vi "Main_flow_full_mqtt_correct.vi"() -> ()   [LabVIEW 2022 SP3]
uses:
  D:/UOM/EE2044 - Electrical Measurements and Instrumentation/Project/Measurment Project/Quaxo_MQTT_LabVIEW-master/Controls/Connection_Return_Codes.ctl
  D:/UOM/EE2044 - Electrical Measurements and Instrumentation/Project/Measurment Project/Quaxo_MQTT_LabVIEW-master/Controls/QoS.ctl
  D:/UOM/EE2044 - Electrical Measurements and Instrumentation/Project/Measurment Project/Quaxo_MQTT_LabVIEW-master/Controls/Retain_Flag.ctl
  D:/UOM/EE2044 - Electrical Measurements and Instrumentation/Project/Measurment Project/Quaxo_MQTT_LabVIEW-master/Controls/DUP_Flag.ctl
  D:/UOM/EE2044 - Electrical Measurements and Instrumentation/Project/Measurment Project/Quaxo_MQTT_LabVIEW-master/Controls/Connect_Flags.ctl
  D:/UOM/EE2044 - Electrical Measurements and Instrumentation/Project/Measurment Project/Quaxo_MQTT_LabVIEW-master/Controls/User_Info.ctl
  <vilib>/DAQmx/write.llb/DAQmx Write (Digital Bool 1Line 1Point).vi
  <vilib>/DAQmx/read.llb/DAQmx Read (Digital Bool 1Line 1Point).vi
  <vilib>/DAQmx/read.llb/DAQmx Read (Analog 1D DBL NChan 1Samp).vi
  <vilib>/DAQmx/create/channels.llb/DAQmx Create Channel (AI-Voltage-Basic).vi
  <vilib>/DAQmx/create/channels.llb/DAQmx Create Channel (DO-Digital Output).vi
  <vilib>/DAQmx/create/channels.llb/DAQmx Create Channel (DI-Digital Input).vi
  <vilib>/DAQmx/miscellaneous.llb/DAQmx Fill In Error Info.vi
  D:/UOM/EE2044 - Electrical Measurements and Instrumentation/Project/Measurment Project/Quaxo_MQTT_LabVIEW-master/MQTT_Functions.lvlib
panel:
  out "?":bool
  out "?":bool
  out "?":bool
  in  "stop 2":bool
  in  "Publish Meta":cluster{"QoS":T1, "Retain":T2, "DUP":T3}
  out "Connection Status":T4=enum."Connection refused: not authorized"
  in  "MQTT Broker":cluster{"address (IP)":string, "port":u16}={"address (IP)"="broker.mqttdashboard.com", "port"=1883}
  in  "Client ID":string="NodeE-12345"
  out "main loop executed":dbl
  out "Servo Angle":dbl(knob) scale=0.0..150.0
  in  "stop (F)":bool
  out "PWM Wave":dynamicdata(graph) caption="Square"
  in  "Frequency":dbl=50.0
  in  "Offset":dbl=2.5
  in  "Amplitude":dbl=2.5
  out "LDR Value":dbl(knob) scale=0.0..10.0
  in  "Relay 2":tag
  in  "Relay 1":tag
  in  "UP DOWN 2":tag
  in  "UP DOWN 1":tag
  in  "Buzzer":tag
  out "Counter":dbl
  out "OUT COUNT":dbl
  out "IN COUNT":dbl
  in  "Door IR 1 & 2 & LDR":tag
  in  "Trigger Period(sec)":dbl
  out "Current Time":dbl
  in  "Mode":dbl
  in  "stop":bool
  # "Light Mode"
  # "Dev1/ai4:6"
  # "Low"
  # "Medium"
  # "High"
  # "Dev1/port0/line2"
  # "This Indicate the status of light mode in the room"
  # "Dev1/port0/line0"
  # "Dev1/port0/line1"
  # "Dev1/port0/line3"
  # "Dev1/port0/line4"
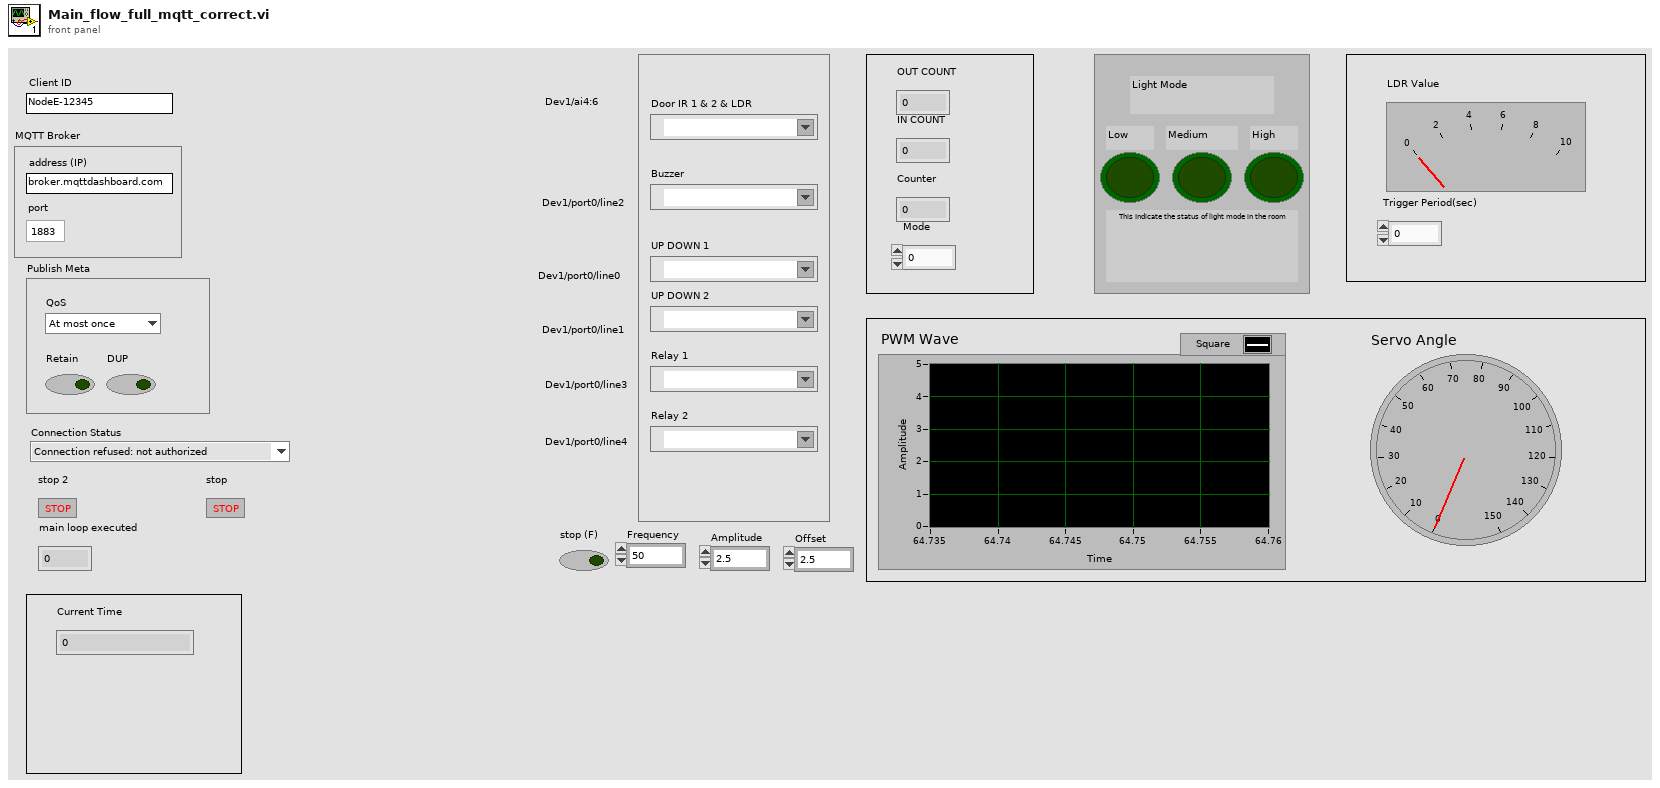
[diagram p1: front panel]
types:
  T1 = typedef "MQTT_Functions.lvlib/QoS.ctl" = enum8{"At most once", "At least once", "Exactly once", "Reserved"}
  T2 = typedef "MQTT_Functions.lvlib/Retain_Flag.ctl" = bool
  T3 = typedef "MQTT_Functions.lvlib/DUP_Flag.ctl" = bool
  T4 = typedef "MQTT_Functions.lvlib/Connection_Return_Codes.ctl" = enum16{"Connection accepted", "Connection refused: unacceptable protocol version", "Connection refused: identifier rejected", "Connection refused: Server unavailable", "Connection refused: bad user name or password", "Connection refused: not authorized"}
  T5 = typedef "MQTT_Functions.lvlib/User_Info.ctl" = cluster{"User Name":string, "Password":string}
  T6 = typedef "MQTT_Functions.lvlib/Connect_Flags.ctl" = cluster{"user name":bool, "password":bool, "will retain":bool, "will flag":bool, "clean session":bool, "reserved":bool, "will QoS":T1}
  T7 = cluster{"QoS":T1, "DUP":T3, "Retain":T2, "Keep Alive (sec)":u16}
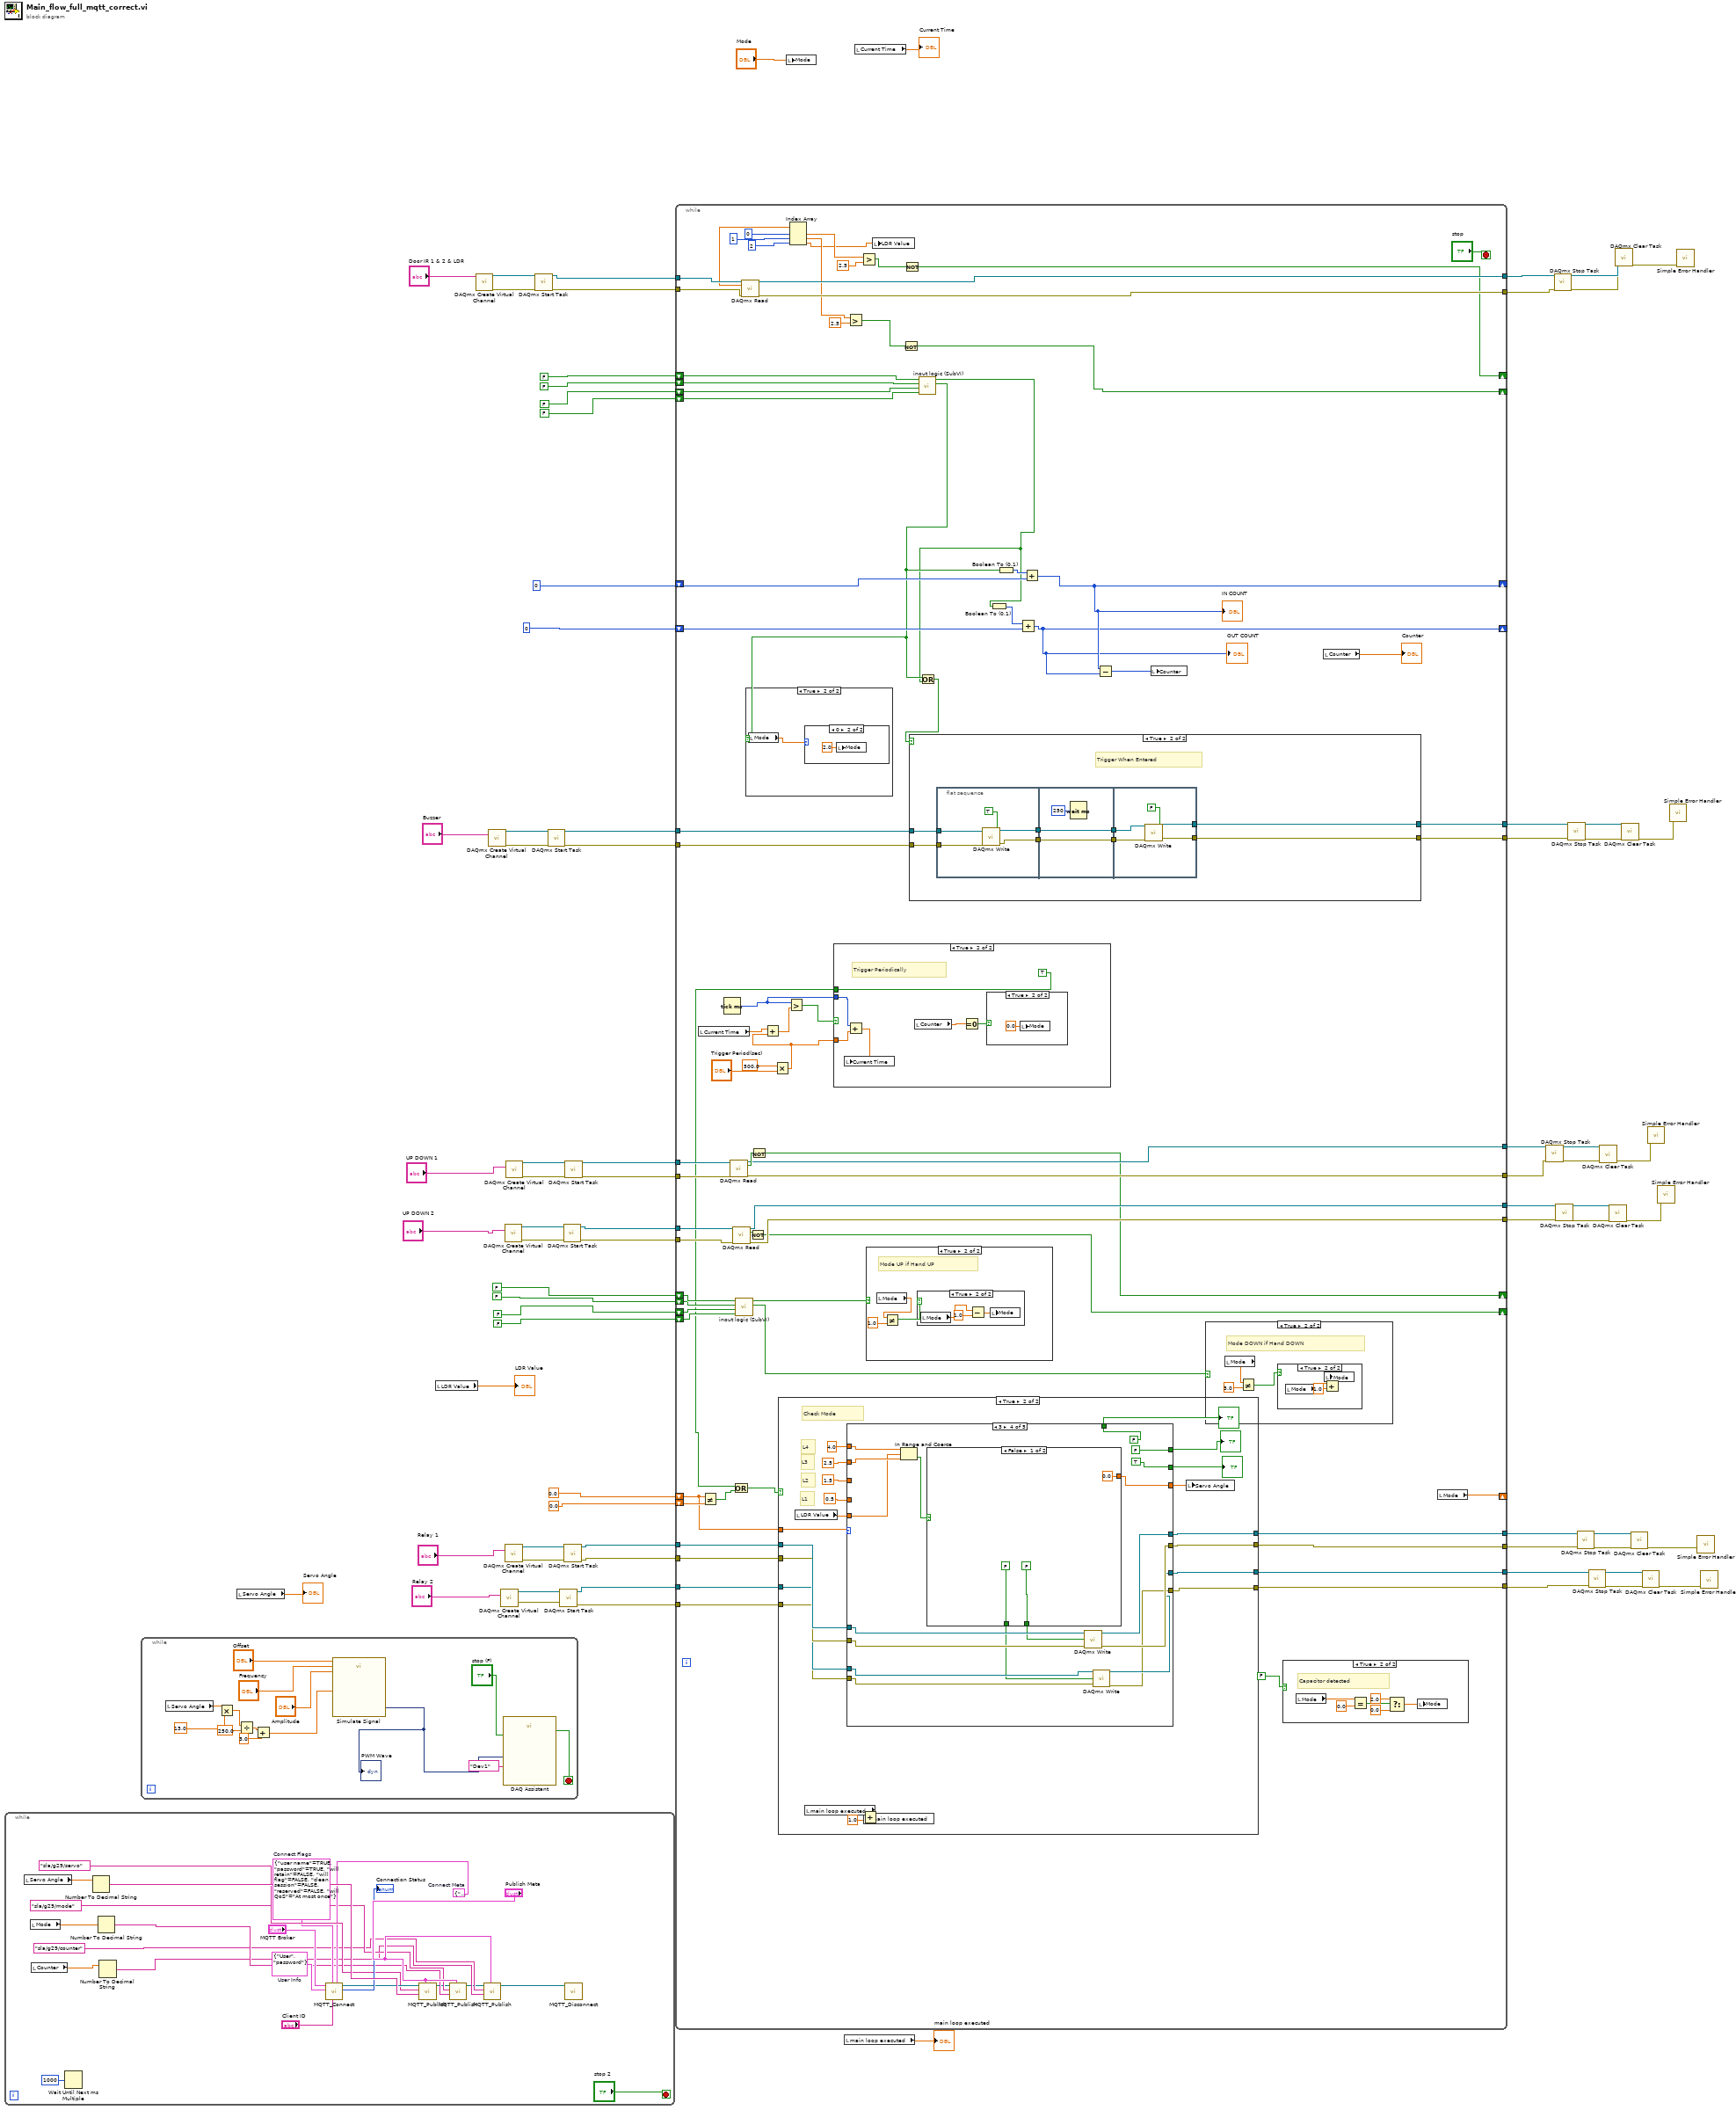
[diagram p0: block diagram]
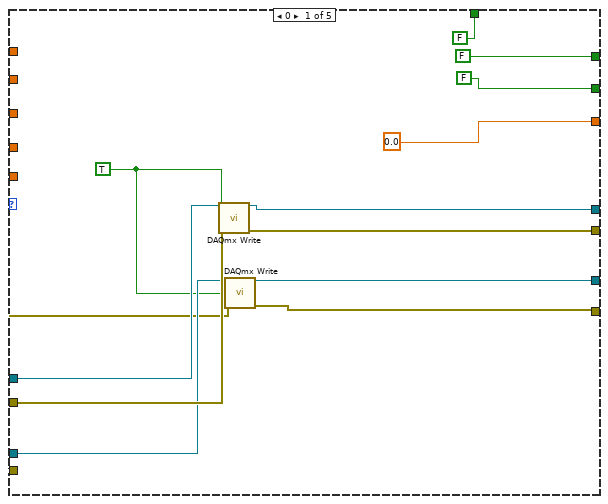
[diagram p5: hidden frame]
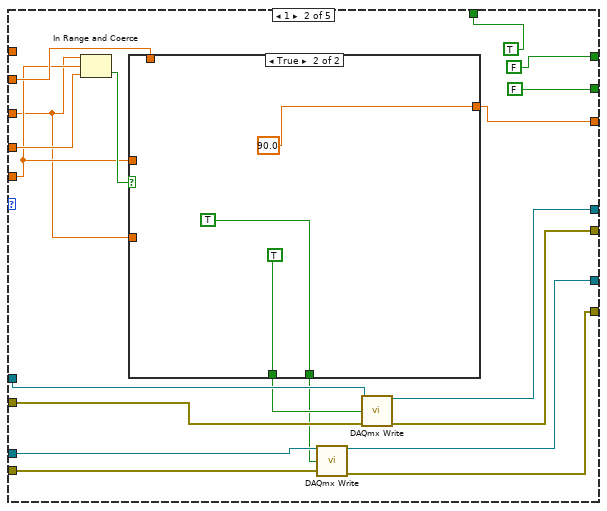
[diagram p6: hidden frame]
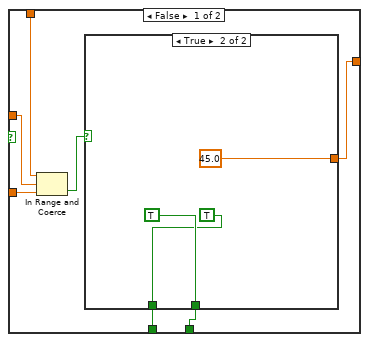
[diagram p7: hidden frame]
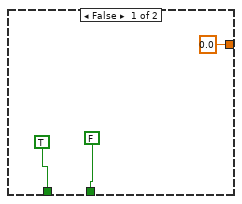
[diagram p8: hidden frame]
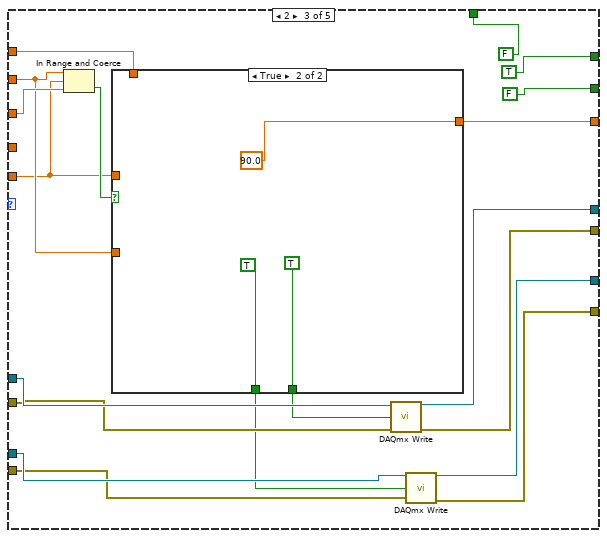
[diagram p9: hidden frame]
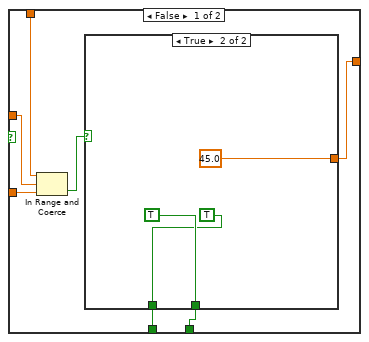
[diagram p10: hidden frame]
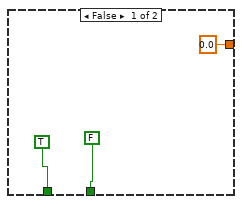
[diagram p11: hidden frame]
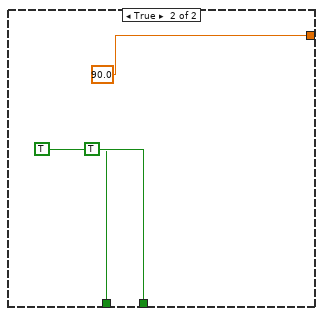
[diagram p12: hidden frame]
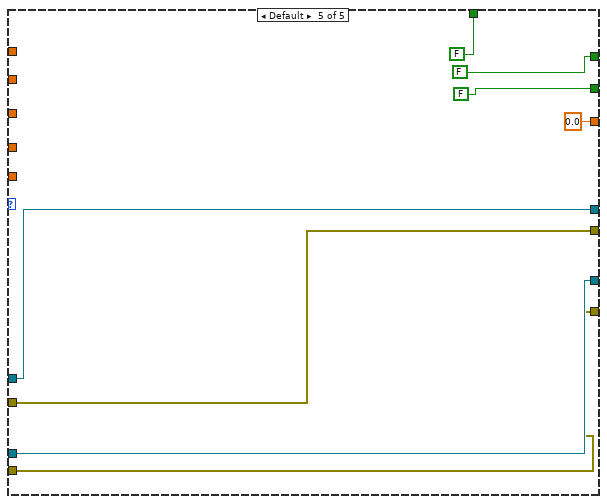
[diagram p13: hidden frame]
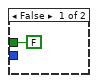
[diagram p18: hidden frame]
diagram:
  n1 = while {
    stop <- "stop 2" stop-if-true
    w85 = T5 {"User Name"="User", "Password"="password"}  # User Info
    w86 = T6 {"user name"=TRUE, "password"=TRUE, "will retain"=FALSE, "will flag"=FALSE, "clean session"=FALSE, "reserved"=FALSE, "will QoS"=enum."At most once"}  # Connect Flags
    w87 = T7 {"QoS"=enum."At most once", "DUP"=FALSE, "Retain"=FALSE, "Keep Alive (sec)"=60}  # Connect Meta
    n2 = local read "Servo Angle"() -> (w96:dbl)
    n3 = local read "Mode"() -> (w98:dbl)
    n4 = local read "Counter"() -> (w97:dbl)
    n5 = Wait Until Next ms Multiple(millisecond multiple=u32 1000) -> ()  [unwired: 1 out]
    n6 = Number To Decimal String(number=w96) -> (decimal integer string=w95:string)  [unwired: 1 in]
    n7 = Number To Decimal String(number=w98) -> (decimal integer string=w84:string)  [unwired: 1 in]
    n8 = Number To Decimal String(number=w97) -> (decimal integer string=w82:string)  [unwired: 1 in]
    n9 = call "MQTT_Connect.vi"("Connect Meta"=w87, "Client ID"="Client ID", "Connect Flags"=w86, "User Info"=w85, "MQTT Broker"="MQTT Broker") -> ("Connection Status"=→"Connection Status":T4, "connection ID out"=w92:refnum<k5>)  [unwired: 4 in, 1 out]
    n10 = call "MQTT_Publish.vi"("Publish Meta"="Publish Meta", "Message to be published"=w95, "Topic"="sla/g29/servo", "connection ID"=w92) -> ("connection ID out"=w79:refnum<k5>)  [unwired: 6 in, 1 out]
    n11 = call "MQTT_Publish.vi"("Publish Meta"="Publish Meta", "Message to be published"=w84, "Topic"="sla/g29/mode", "connection ID"=w79) -> ("connection ID out"=w78:refnum<k5>)  [unwired: 6 in, 1 out]
    n12 = call "MQTT_Publish.vi"("Publish Meta"="Publish Meta", "Message to be published"=w82, "Topic"="sla/g29/counter", "connection ID"=w78) -> ("connection ID out"=w90:refnum<k5>)  [unwired: 6 in, 1 out]
    n13 = call "MQTT_Disconnect.vi"("connection ID"=w90) -> ()  [unwired: 10 in, 1 out]
  }
  n14 = while {
    stop <- w112 stop-if-true
    n15 = local read "Servo Angle"() -> (w100:dbl)
    n16 = Multiply(x=w100, y=13.0) -> (x*y=w106:dbl)
    n17 = Divide(x=w106, y=250.0) -> (x/y=w105:dbl)
    n18 = Add(x=w105, y=3.0) -> (x+y=w101:dbl)
    n19 = call "Simulate Signal"("Offset"="Offset", "Duty Cycle (%)"=w101, "Frequency"="Frequency", "Amplitude"="Amplitude") -> ("Square"=w108:dynamicdata)  [unwired: 10 in, 1 out]
    "PWM Wave" <- w108
    n20 = call "DAQ Assistant"("data"=w108, "stop (F)"="stop (F)", "device name"=tag "Dev1") -> ("stopped"=w112:bool)  [unwired: 14 in, 2 out]
  }
  n21 = local read "Servo Angle"() -> (→"Servo Angle":dbl)
  n22 = local read "LDR Value"() -> (→"LDR Value":dbl)
  n23 = call-poly <vilib>:"DAQmx Create Virtual Channel.vi"("physical channels"="Door IR 1 & 2 & LDR") -> ("task out"=w73:refnum<k21>, "error out"=w70:errorcluster)  [unwired: 13 in]
  n24 = call-poly <vilib>:"DAQmx Create Virtual Channel.vi"("lines"="Buzzer") -> ("task out"=w58:refnum<k21>, "error out"=w56:errorcluster)  [unwired: 13 in]
  n25 = call-poly <vilib>:"DAQmx Create Virtual Channel.vi"("lines"="Relay 2") -> ("task out"=w19:refnum<k21>, "error out"=w18:errorcluster)  [unwired: 13 in]
  n26 = call-poly <vilib>:"DAQmx Create Virtual Channel.vi"("lines"="UP DOWN 2") -> ("task out"=w47:refnum<k21>, "error out"=w45:errorcluster)  [unwired: 13 in]
  n27 = call-poly <vilib>:"DAQmx Create Virtual Channel.vi"("lines"="Relay 1") -> ("task out"=w22:refnum<k21>, "error out"=w21:errorcluster)  [unwired: 13 in]
  n28 = call-poly <vilib>:"DAQmx Create Virtual Channel.vi"("lines"="UP DOWN 1") -> ("task out"=w48:refnum<k21>, "error out"=w46:errorcluster)  [unwired: 13 in]
  n29 = call <vilib>:"DAQmx Start Task.vi"("task/channels in"=w73, "error in"=w70) -> ("task out"=w71:refnum<k21>, "error out"=w69:errorcluster)  [unwired: 12 in]
  n30 = call <vilib>:"DAQmx Start Task.vi"("task/channels in"=w58, "error in"=w56) -> ("task out"=w55:refnum<k21>, "error out"=w54:errorcluster)  [unwired: 12 in]
  n31 = call <vilib>:"DAQmx Start Task.vi"("task/channels in"=w19, "error in"=w18) -> ("task out"=w14:refnum<k21>, "error out"=w13:errorcluster)  [unwired: 12 in]
  n32 = call <vilib>:"DAQmx Start Task.vi"("task/channels in"=w47, "error in"=w45) -> ("task out"=w40:refnum<k21>, "error out"=w39:errorcluster)  [unwired: 12 in]
  n33 = call <vilib>:"DAQmx Start Task.vi"("task/channels in"=w22, "error in"=w21) -> ("task out"=w16:refnum<k21>, "error out"=w15:errorcluster)  [unwired: 12 in]
  n34 = call <vilib>:"DAQmx Start Task.vi"("task/channels in"=w48, "error in"=w46) -> ("task out"=w42:refnum<k21>, "error out"=w41:errorcluster)  [unwired: 12 in]
  n35 = while {
    shift-right: [w182] -> _
    shift-left: 0.0 ("Mode") -> [w180]
    shift-left: 0.0 ("Mode") -> [w181]
    tunnel: w71 -> [w177]
    tunnel: w69 -> [w176]
    tunnel: [w175] -> w68
    tunnel: [w174] -> w67
    shift-right: [w165] -> _
    shift-left: FALSE -> [w173]
    shift-left: FALSE -> [w172]
    shift-right: [w168] -> _
    shift-left: FALSE -> [w171]
    shift-left: FALSE -> [w142]
    shift-right: [w167] -> _
    shift-left: 0 -> [w170]
    shift-right: [w166] -> _
    shift-left: 0 -> [w169]
    tunnel: w55 -> [w162]
    tunnel: w54 -> [w161]
    tunnel: [w160] -> w50
    tunnel: [w159] -> w49
    shift-right: [w148] -> _
    shift-left: FALSE -> [w146]
    shift-right: [w147] -> _
    shift-left: FALSE -> [w144]
    shift-left: FALSE -> [w145]
    shift-left: FALSE -> [w143]
    tunnel: w42 -> [w156]
    tunnel: w41 -> [w155]
    tunnel: w40 -> [w154]
    tunnel: w39 -> [w153]
    tunnel: [w152] -> w32
    tunnel: [w151] -> w31
    tunnel: [w150] -> w30
    tunnel: [w149] -> w29
    tunnel: w16 -> [w124]
    tunnel: w15 -> [w123]
    tunnel: w14 -> [w122]
    tunnel: w13 -> [w121]
    tunnel: [w120] -> w6
    tunnel: [w119] -> w5
    tunnel: [w118] -> w4
    tunnel: [w117] -> w3
    stop <- "stop" stop-if-true
    n36 = local read "Current Time"() -> (w189:dbl)
    n37 = Not Equal?(x=w180, y=w181) -> (x != y?=w116:bool)
    n38 = Tick Count (ms)() -> (millisecond timer value=w187:u32)
    n39 = call-poly <vilib>:"DAQmx Read.vi"("task/channels in"=w156, "error in"=w155) -> ("task out"=w152:refnum<k21>, "data"=w158:bool, "error out"=w151:errorcluster)  [unwired: 11 in]
    n40 = call-poly <vilib>:"DAQmx Read.vi"("task/channels in"=w154, "error in"=w153) -> ("task out"=w150:refnum<k21>, "data"=w157:bool, "error out"=w149:errorcluster)  [unwired: 11 in]
    n41 = call "inout logic (SubVI).vi"("Sensor 2 (T-2)"=w143, "Sensor 2 (T-1)"=w144, "Sensor 1 (T-2)"=w145, "Sensor 1 (T-1)"=w146) -> ("IN"=w141:bool, "OUT"=w140:bool)  [unwired: 6 in]
    n42 = call-poly <vilib>:"DAQmx Read.vi"("task/channels in"=w177, "error in"=w176) -> ("task out"=w175:refnum<k21>, "data"=w134:dbl[], "error out"=w174:errorcluster)  [unwired: 11 in]
    n43 = Not(x=w157) -> (.not. x?=w147:bool)
    n44 = Not(x=w158) -> (.not. x?=w148:bool)
    n45 = Multiply(x=500.0, y="Trigger Period(sec)") -> (x*y=w183:dbl)
    n46 = Add(x=w189, y=w183) -> (x+y=w186:dbl)
    n47 = Greater?(x=w187, y=w186) -> (0:w188:bool)
    n48 = Index Array(array=w134, index #1=0 ("index"), index #2=1 ("index"), index #3=2 ("index")) -> (element #1=w133:dbl, element #2=w130:dbl, element #3=w125:dbl)
    n49 = case shown="True" w188 {
      tunnel: w187 -> [_ w350]
      tunnel: w183 -> [_ w349]
      tunnel: [FALSE ("Check") TRUE ("Check")] -> w114
      frame False {
      }
      frame True {
        # "Trigger Periodically"
        n50 = Add(x=w350, y=w349) -> (x+y=w351:dbl)
        n51 = local write "Current Time"(w351) -> ()
        n52 = local read "Counter"() -> (w348:dbl)
        n53 = Equal To 0?(x=w348) -> (x = 0?=w347:bool)
        n54 = case shown="True" w347 {
          frame False {
          }
          frame True {
            n55 = local write "Mode"(0.0 ("Mode")) -> ()
          }
        }
      }
    }
    n56 = Or(x=w114, y=w116) -> (x .or. y?=w115:bool)
    n57 = case shown="True" w115 {
      tunnel: w180 -> [_ w217]
      tunnel: w124 -> [w196 w216]
      tunnel: w123 -> [w195 w215]
      tunnel: w122 -> [w194 w214]
      tunnel: w121 -> [w193 w213]
      tunnel: [w196 w212] -> w120
      tunnel: [w195 w211] -> w119
      tunnel: [w194 w210] -> w118
      tunnel: [w193 w209] -> w117
      frame False {
      }
      frame True {
        # "L4"
        # "L1"
        # "L3"
        # "L2"
        # "Check Mode"
        n58 = local read "LDR Value"() -> (w207:dbl)
        n59 = local read "main loop executed"() -> (w202:dbl)
        n60 = case shown="3" w217 {
          tunnel: w216 -> [w230 w249 w284 w318 w332]
          tunnel: w215 -> [w229 w247 w283 w317 w331]
          tunnel: w214 -> [w228 w245 w282 w316 w330]
          tunnel: w213 -> [w227 w243 w281 w315 w329]
          tunnel: [w226 w248 w280 w314 w332] -> w212
          tunnel: [w225 w246 w279 w313 w331] -> w211
          tunnel: [w224 w244 w278 w312 w330] -> w210
          tunnel: [w223 w242 w277 w311 w329] -> w209
          tunnel: 1.5 -> [_ w237 w276 _ _]
          tunnel: 0.5 -> [_ w240 _ _ _]
          tunnel: w207 -> [_ w238 w269 w307 _]
          tunnel: 2.5 -> [_ w239 w270 w308 _]
          tunnel: 4.0 -> [_ _ w271 w309 _]
          tunnel: [0.0 ("Servo Angle") w234 w274 w306 0.0 ("A")] -> w203
          tunnel: [FALSE TRUE FALSE FALSE FALSE] -> w199
          tunnel: [FALSE FALSE TRUE FALSE FALSE] -> w198
          tunnel: [FALSE FALSE FALSE TRUE FALSE] -> w197
          frame 0 {
            w222 = TRUE ("data")
            n61 = call-poly <vilib>:"DAQmx Write.vi"("task/channels in"=w230, "data"=w222, "error in"=w229) -> ("task out"=w226:refnum<k21>, "error out"=w225:errorcluster)  [unwired: 10 in, 1 out]
            n62 = call-poly <vilib>:"DAQmx Write.vi"("task/channels in"=w228, "data"=w222, "error in"=w227) -> ("task out"=w224:refnum<k21>, "error out"=w223:errorcluster)  [unwired: 10 in, 1 out]
          }
          frame 1 {
            n63 = In Range and Coerce(upper limit=w237, x=w238, lower limit=w240) -> (In Range?=w241:bool)  [unwired: 1 out]
            n64 = case shown="True" w241 {
              tunnel: [w252 90.0] -> w234
              tunnel: [w251 TRUE] -> w235
              tunnel: [w250 TRUE] -> w236
              tunnel: w239 -> [w256 _]
              tunnel: w237 -> [w255 _]
              tunnel: w238 -> [w254 _]
              frame False {
                n65 = In Range and Coerce(upper limit=w256, x=w254, lower limit=w255) -> (In Range?=w253:bool)  [unwired: 1 out]
                n66 = case shown="True" w253 {
                  tunnel: [0.0 45.0] -> w252
                  tunnel: [FALSE TRUE] -> w251
                  tunnel: [TRUE TRUE] -> w250
                  frame False {
                  }
                  frame True {
                  }
                }
              }
              frame True {
              }
            }
            n67 = call-poly <vilib>:"DAQmx Write.vi"("task/channels in"=w245, "data"=w235, "error in"=w243) -> ("task out"=w244:refnum<k21>, "error out"=w242:errorcluster)  [unwired: 10 in, 1 out]
            n68 = call-poly <vilib>:"DAQmx Write.vi"("task/channels in"=w249, "data"=w236, "error in"=w247) -> ("task out"=w248:refnum<k21>, "error out"=w246:errorcluster)  [unwired: 10 in, 1 out]
          }
          frame 2 {
            n69 = In Range and Coerce(upper limit=w270, x=w269, lower limit=w276) -> (In Range?=w275:bool)  [unwired: 1 out]
            n70 = case shown="True" w275 {
              tunnel: [w287 90.0] -> w274
              tunnel: [w286 TRUE] -> w273
              tunnel: [w285 TRUE] -> w272
              tunnel: w271 -> [w291 _]
              tunnel: w270 -> [w290 _]
              tunnel: w269 -> [w289 _]
              frame False {
                n71 = In Range and Coerce(upper limit=w291, x=w289, lower limit=w290) -> (In Range?=w288:bool)  [unwired: 1 out]
                n72 = case shown="True" w288 {
                  tunnel: [0.0 45.0] -> w287
                  tunnel: [FALSE TRUE] -> w286
                  tunnel: [TRUE TRUE] -> w285
                  frame False {
                  }
                  frame True {
                  }
                }
              }
              frame True {
              }
            }
            n73 = call-poly <vilib>:"DAQmx Write.vi"("task/channels in"=w284, "data"=w273, "error in"=w283) -> ("task out"=w280:refnum<k21>, "error out"=w279:errorcluster)  [unwired: 10 in, 1 out]
            n74 = call-poly <vilib>:"DAQmx Write.vi"("task/channels in"=w282, "data"=w272, "error in"=w281) -> ("task out"=w278:refnum<k21>, "error out"=w277:errorcluster)  [unwired: 10 in, 1 out]
          }
          frame 3 {
            n75 = In Range and Coerce(upper limit=w309, x=w307, lower limit=w308) -> (In Range?=w310:bool)  [unwired: 1 out]
            n76 = case shown="False" w310 {
              tunnel: [0.0 90.0] -> w306
              tunnel: [FALSE TRUE] -> w305
              tunnel: [FALSE TRUE] -> w304
              frame False {
              }
              frame True {
              }
            }
            n77 = call-poly <vilib>:"DAQmx Write.vi"("task/channels in"=w318, "data"=w305, "error in"=w317) -> ("task out"=w314:refnum<k21>, "error out"=w313:errorcluster)  [unwired: 10 in, 1 out]
            n78 = call-poly <vilib>:"DAQmx Write.vi"("task/channels in"=w316, "data"=w304, "error in"=w315) -> ("task out"=w312:refnum<k21>, "error out"=w311:errorcluster)  [unwired: 10 in, 1 out]
          }
          frame Default {
          }
        }
        "?" <- w197
        "?" <- w198
        "?" <- w199
        n79 = Add(x=w202, y=1.0) -> (x+y=w200:dbl)
        n80 = local write "main loop executed"(w200) -> ()
        n81 = local write "Servo Angle"(w203) -> ()
      }
    }
    n82 = Greater?(x=w130, y=2.5) -> (0:w136:bool)
    n83 = Greater?(x=w133, y=2.5) -> (0:w138:bool)
    n84 = case shown="True" w140 {
      frame False {
      }
      frame True {
        # "Mode UP if Hand UP"
        n85 = local read "Mode"() -> (w335:dbl)
        n86 = Not Equal?(x=w335, y=1.0) -> (x != y?=w334:bool)
        n87 = case shown="True" w334 {
          frame False {
          }
          frame True {
            n88 = local read "Mode"() -> (w337:dbl)
            n89 = Subtract(x=w337, y=1.0) -> (x-y=w336:dbl)
            n90 = local write "Mode"(w336) -> ()
          }
        }
      }
    }
    n91 = local write "LDR Value"(w125) -> ()
    n92 = Not(x=w136) -> (.not. x?=w168:bool)
    n93 = Not(x=w138) -> (.not. x?=w165:bool)
    n94 = call "inout logic (SubVI).vi"("Sensor 2 (T-2)"=w142, "Sensor 2 (T-1)"=w171, "Sensor 1 (T-2)"=w172, "Sensor 1 (T-1)"=w173) -> ("IN"=w129:bool, "OUT"=w128:bool)  [unwired: 6 in]
    n95 = case shown="True" w129 {
      frame False {
      }
      frame True {
        n96 = local read "Mode"() -> (w191:dbl)
        n97 = case shown="0" w191 {
          frame Default {
          }
          frame 0 {
            n98 = local write "Mode"(2.0 ("Mode")) -> ()
          }
        }
      }
    }
    n99 = Or(x=w129, y=w128) -> (x .or. y?=w127:bool)
    n100 = case shown="True" w127 {
      tunnel: w162 -> [w353 w362]
      tunnel: w161 -> [w354 w361]
      tunnel: [w353 w356] -> w160
      tunnel: [w354 w355] -> w159
      frame False {
      }
      frame True {
        # "Trigger When Entered"
        n101 = flat-sequence {
          tunnel: w362 -> [w366]
          tunnel: w361 -> [w365]
          tunnel: [w364] -> w359
          tunnel: [w363] -> w357
          tunnel: [w369] -> w360
          tunnel: w359 -> [w369]
          tunnel: [w368] -> w358
          tunnel: w357 -> [w368]
          tunnel: w360 -> [w374]
          tunnel: w358 -> [w373]
          tunnel: [w372] -> w356
          tunnel: [w371] -> w355
          frame #0 {
            n102 = call-poly <vilib>:"DAQmx Write.vi"("task/channels in"=w366, "data"=TRUE, "error in"=w365) -> ("task out"=w364:refnum<k21>, "error out"=w363:errorcluster)  [unwired: 10 in, 1 out]
          }
          frame #1 {
            n103 = Wait (ms)(milliseconds to wait=u32 250) -> ()  [unwired: 1 out]
          }
          frame #2 {
            n104 = call-poly <vilib>:"DAQmx Write.vi"("task/channels in"=w374, "data"=FALSE, "error in"=w373) -> ("task out"=w372:refnum<k21>, "error out"=w371:errorcluster)  [unwired: 10 in, 1 out]
          }
        }
      }
    }
    n105 = Boolean To (0,1)(Boolean=w128) -> (0, 1=w178:i16)
    n106 = Boolean To (0,1)(Boolean=w129) -> (0, 1=w179:i16)
    n107 = Add(x=w178, y=w169) -> (x+y=w166:i32)
    "OUT COUNT" <- w166
    n108 = Add(x=w179, y=w170) -> (x+y=w167:i32)
    "IN COUNT" <- w167
    n109 = Subtract(x=w167, y=w166) -> (x-y=w164:i32)
    n110 = local write "Counter"(w164) -> ()
    n111 = case shown="True" w141 {
      frame False {
      }
      frame True {
        # "Mode DOWN if Hand DOWN"
        n112 = local read "Mode"() -> (w341:dbl)
        n113 = Not Equal?(x=w341, y=3.0) -> (x != y?=w339:bool)
        n114 = case shown="True" w339 {
          frame False {
          }
          frame True {
            n115 = local read "Mode"() -> (w344:dbl)
            n116 = Add(x=w344, y=1.0) -> (x+y=w342:dbl)
            n117 = local write "Mode"(w342) -> ()
          }
        }
      }
    }
    n118 = case shown="True" FALSE {
      frame False {
      }
      frame True {
        # "Capacitor detected"
        n119 = local read "Mode"() -> (w381:dbl)
        n120 = Equal?(x=w381, y=0.0) -> (x = y?=w379:bool)
        n121 = Select(t=2.0, s=w379, f=0.0) -> (s? t:f=w378:dbl)
        n122 = local write "Mode"(w378) -> ()
      }
    }
    n123 = local read "Counter"() -> (→"Counter":dbl)
    n124 = local read "Mode"() -> (w182:dbl)
  }
  n125 = local write "Mode"("Mode") -> ()
  n126 = local read "main loop executed"() -> (→"main loop executed":dbl)
  n127 = local read "Current Time"() -> (→"Current Time":dbl)
  n128 = call <vilib>:"DAQmx Stop Task.vi"("task/channels in"=w32, "error in"=w31) -> ("task out"=w38:refnum<k21>, "error out"=w36:errorcluster)  [unwired: 12 in]
  n129 = call <vilib>:"DAQmx Stop Task.vi"("task/channels in"=w68, "error in"=w67) -> ("task out"=w66:refnum<k21>, "error out"=w65:errorcluster)  [unwired: 12 in]
  n130 = call <vilib>:"DAQmx Stop Task.vi"("task/channels in"=w30, "error in"=w29) -> ("task out"=w35:refnum<k21>, "error out"=w33:errorcluster)  [unwired: 12 in]
  n131 = call <vilib>:"DAQmx Stop Task.vi"("task/channels in"=w50, "error in"=w49) -> ("task out"=w53:refnum<k21>, "error out"=w51:errorcluster)  [unwired: 12 in]
  n132 = call <vilib>:"DAQmx Stop Task.vi"("task/channels in"=w6, "error in"=w5) -> ("task out"=w12:refnum<k21>, "error out"=w10:errorcluster)  [unwired: 12 in]
  n133 = call <vilib>:"DAQmx Stop Task.vi"("task/channels in"=w4, "error in"=w3) -> ("task out"=w9:refnum<k21>, "error out"=w7:errorcluster)  [unwired: 12 in]
  n134 = call <vilib>:"DAQmx Clear Task.vi"("task in"=w38, "error in"=w36) -> ("error out"=w37:errorcluster)  [unwired: 13 in]
  n135 = call <vilib>:"DAQmx Clear Task.vi"("task in"=w35, "error in"=w33) -> ("error out"=w34:errorcluster)  [unwired: 13 in]
  n136 = call <vilib>:"DAQmx Clear Task.vi"("task in"=w66, "error in"=w65) -> ("error out"=w64:errorcluster)  [unwired: 13 in]
  n137 = call <vilib>:"DAQmx Clear Task.vi"("task in"=w53, "error in"=w51) -> ("error out"=w52:errorcluster)  [unwired: 13 in]
  n138 = call <vilib>:"DAQmx Clear Task.vi"("task in"=w12, "error in"=w10) -> ("error out"=w11:errorcluster)  [unwired: 13 in]
  n139 = call <vilib>:"DAQmx Clear Task.vi"("task in"=w9, "error in"=w7) -> ("error out"=w8:errorcluster)  [unwired: 13 in]
  n140 = call <vilib>:"Simple Error Handler.vi"("error in (no error)"=w37) -> ()  [unwired: 4 in, 5 out]
  n141 = call <vilib>:"Simple Error Handler.vi"("error in (no error)"=w34) -> ()  [unwired: 4 in, 5 out]
  n142 = call <vilib>:"Simple Error Handler.vi"("error in (no error)"=w52) -> ()  [unwired: 4 in, 5 out]
  n143 = call <vilib>:"Simple Error Handler.vi"("error in (no error)"=w64) -> ()  [unwired: 4 in, 5 out]
  n144 = call <vilib>:"Simple Error Handler.vi"("error in (no error)"=w11) -> ()  [unwired: 4 in, 5 out]
  n145 = call <vilib>:"Simple Error Handler.vi"("error in (no error)"=w8) -> ()  [unwired: 4 in, 5 out]
